vi "AlliGator FMB Run Script.vi"(8 "Error In":errorcluster, 9 "# Steps":i32, 11 "FMB Q Elements in":T18[](array[typedef])) -> (0 "Error Out":errorcluster, 1 "Array of Simulation Outputs":T1[](array[typedef]) {"Simulation & Fit Options & Parameters"."Decay Fit Options & Parameters"."Fit Options"."Confidence Level" min=0.0 max=100.0; "Simulation & Fit Options & Parameters"."Decay Fit Options & Parameters"."Fit Options"."Offset Resolution" min=0.0; "Simulation & Fit Options & Parameters"."Decay Fit Options & Parameters"."Fit Options"."Period" min=0.0; "Simulation & Fit Options & Parameters"."Decay Fit Options & Parameters"."Fit Options"."Min Decay Percentile" min=0.0 max=1.0; "Simulation & Fit Options & Parameters"."Decay Fit Options & Parameters"."Fit Options"."Max Decay Percentile" min=0.0 max=100.0; "Simulation & Fit Options & Parameters"."Decay Fit Options & Parameters"."Fit Parameter Constraints"."Max Value" format="%#.3g"; "Simulation & Fit Options & Parameters"."Decay Fit Options & Parameters"."Fit Parameter Constraints"."Min Value" format="%#.3g"}, 3 "FMB Q Elements out":T18[](array[typedef]), 4 "Message":string)   [LabVIEW 2021, in "AlliGator Fit Method Benchmark.lvlib"]
uses:
  AlliGator Fit Method Benchmark.lvlib
  AlliGator FMB Q Element.ctl
  AlliGator FMB Q Event List.ctl
  Strings/Strings.lvlib
  AlliGator Decay Simulation Parameters.ctl
  AlliGator Fit Simulation Parameters.ctl
  AlliGator Simulation Parameters.ctl
  Fits/Decay Convolution/Decay Model.ctl
  Fits/Fits.lvlib
  Fits/Residual Type.ctl
  Fits/IRF(X)PSED/Fit Weights Type.ctl
  Fits/Non-linear Fitting Method v2.ctl
  Fits/Fit Calculation Method.ctl
  Fits/Non-linear Fitting Algorithm.ctl
  Fits/IRF(X)PSED/Decay Fit Options v3.ctl
  Fits/IRF(X)PSED/Decay Fit Parameters In List.ctl
  Decay Analysis/Decay Fit/AlliGator Decay Fit Parameter Constraints 2.ctl
  Decay Analysis/Decay Fit/AlliGator Decay Fit.lvlib
  Fits/IRF(X)PSED/MLE Baseline Offset Type.ctl
  Decay Fit Parameter Map/AlliGator Decay Fit Options & Parameters v3.ctl
  Decay Fit Parameter Map/AlliGator Decay Fit Parameter Map.lvlib
  AlliGator Simulation & Fit Options & Parameters.ctl
  Arrays/Array Statistics.ctl
  Arrays/Arrays.lvlib
  AlliGator FMB Output.ctl
panel:
  # "see the License on the block diagram (Ctrl+E or Window:Show Block Diagram)"
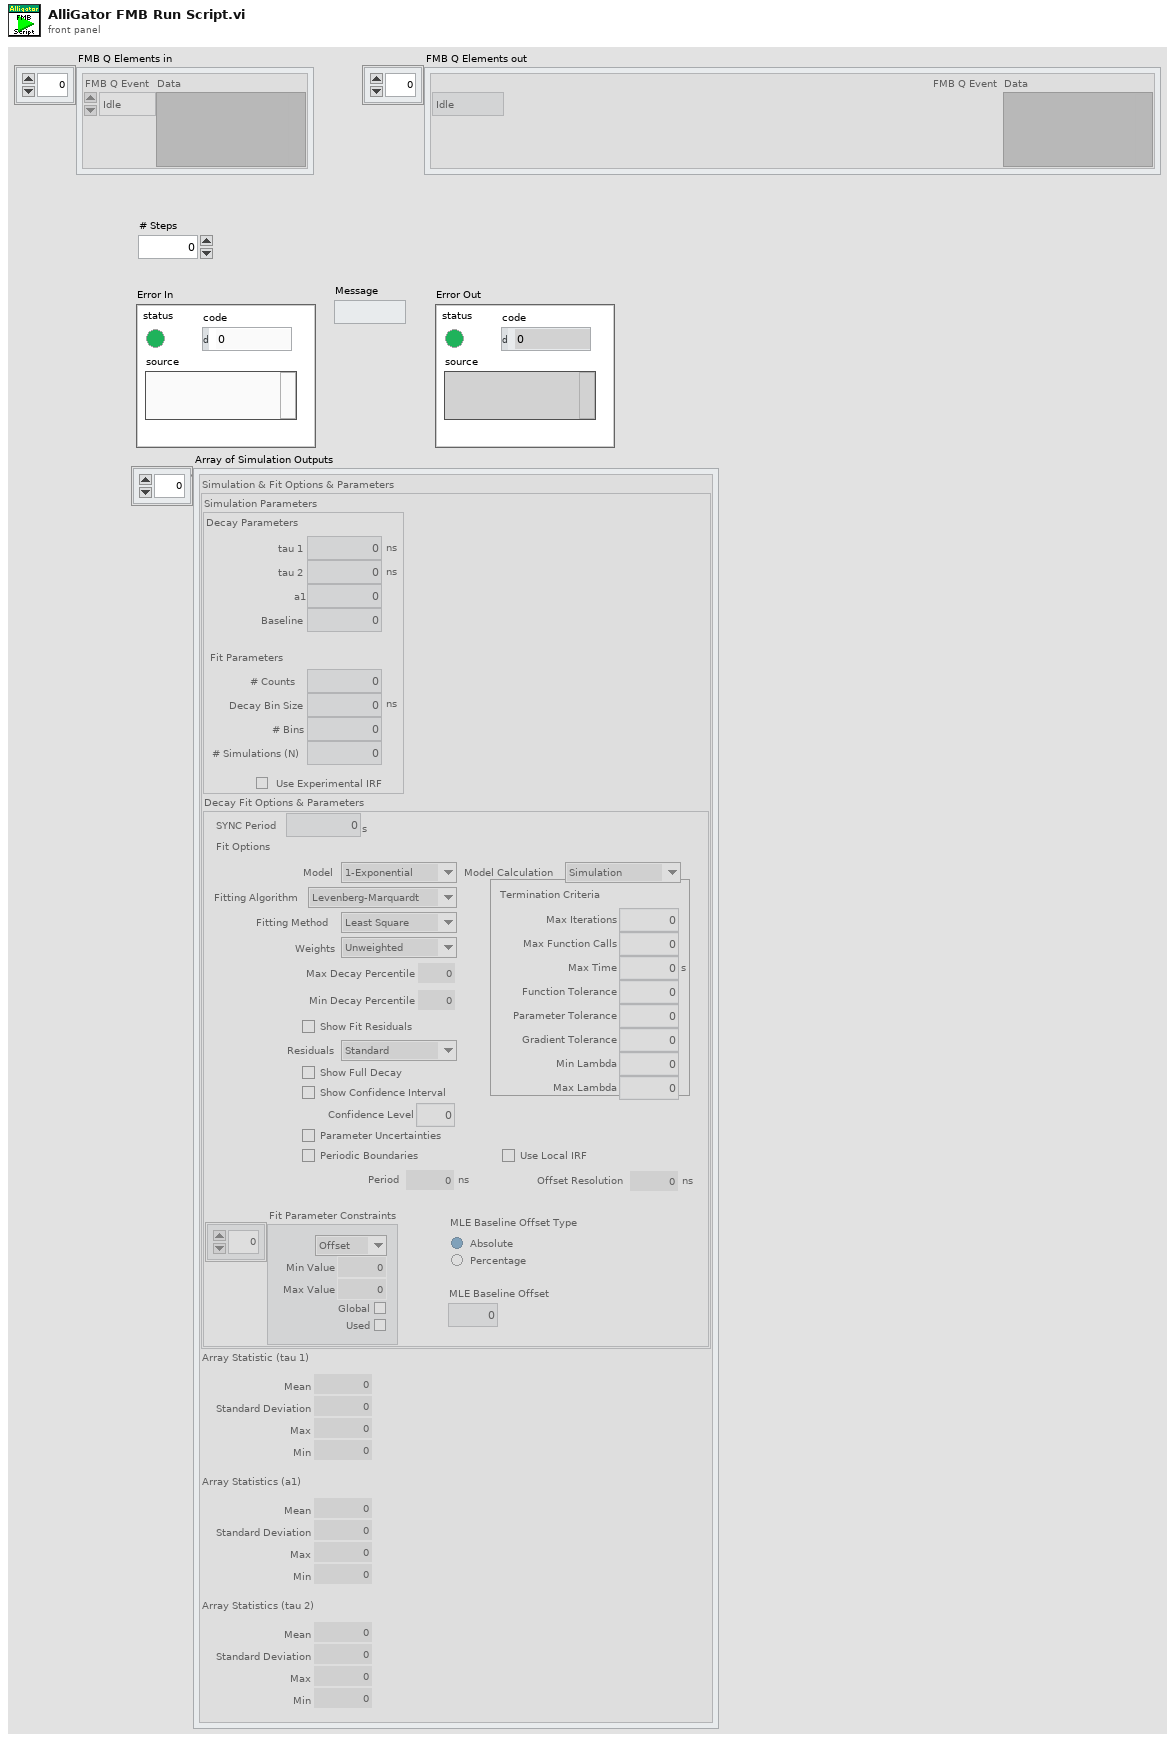
[diagram p1: front panel]
types:
  T1 = typedef "AlliGator Fit Method Benchmark.lvlib/AlliGator FMB Output.ctl" = cluster{"Simulation & Fit Options & Parameters":T2, "Array Statistic (tau 1)":T17, "Array Statistics (a1)":T17, "Array Statistics (tau 2)":T17}
  T2 = typedef "AlliGator Fit Method Benchmark.lvlib/AlliGator Simulation & Fit Options & Parameters.ctl" = cluster{"Simulation Parameters":T3, "Decay Fit Options & Parameters":T6}
  T3 = typedef "AlliGator Fit Method Benchmark.lvlib/AlliGator Simulation Parameters.ctl" = cluster{"Decay Simulation Parameters":T4, "Fit Simulation Parameters":T5, "Use Experimental IRF":bool}
  T4 = typedef "AlliGator Fit Method Benchmark.lvlib/AlliGator Decay Simulation Parameters.ctl" = cluster{"tau 1":dbl[unit], "tau 2":dbl[unit], "a1":dbl, "Baseline":dbl}
  T5 = typedef "AlliGator Fit Method Benchmark.lvlib/AlliGator Fit Simulation Parameters.ctl" = cluster{"# Counts":i32, "# Simulations (N)":i32, "Decay Bin Size":dbl[unit], "# Bins":i32}
  T6 = typedef "AlliGator Decay Fit Parameter Map.lvlib/AlliGator Decay Fit Options & Parameters v3.ctl" = cluster{"SYNC Period":dbl[unit], "Fit Options":T7, "Fit Parameter Constraints":T14[], "MLE Baseline Offset":dbl, "MLE Baseline Offset Type":T16}
  T7 = typedef "Fits.lvlib/Decay Fit Options v3.ctl" = cluster{"Show Fit Residuals":bool, "Fit Model":T8, "Residual Type":T9, "Max Decay Percentile":dbl, "Min Decay Percentile":dbl, "Show Full Decay":bool, "Weights":T10, "Fitting Method":T11, "Compute Parameter Uncertainties":bool, "Periodic Boundaries":bool, "Model Calculation":T12, "Period":dbl[unit], "Termination Criteria":cluster{"Max Iterations":i32, "Max Function Calls":i32, "Max Time":dbl[unit], "Function Tolerance":dbl, "Parameter Tolerance":dbl, "Gradient Tolerance":dbl, "Min Lambda":dbl, "Max Lambda":dbl, "Initial Tick Count":u32}, "Offset Resolution":dbl[unit], "Use Local IRF":bool, "Fitting Algorithm":T13, "Show Confidence Interval ":bool, "Confidence Level":dbl}
  T8 = typedef "Fits.lvlib/Decay Model.ctl" = enum16{"1-Exponential", "2-Exponentials"}
  T9 = typedef "Fits.lvlib/Residual Type.ctl" = enum16{"Standard", "Normalized", "Reduced"}
  T10 = typedef "Fits.lvlib/Fit Weights Type.ctl" = enum16{"Unweighted", "1/Variance", "Best of All"}
  T11 = typedef "Fits.lvlib/Non-linear Fitting Method v2.ctl" = enum16{"Least Square", "Least Absolute Residual", "Bisquare", "MLE", "-", "Best of All"}
  T12 = typedef "Fits.lvlib/Fit Calculation Method.ctl" = enum16{"Simulation", "Convolution", "Integration"}
  T13 = typedef "Fits.lvlib/Non-linear Fitting Algorithm.ctl" = enum16{"Levenberg-Marquardt", "Trust-Region Dogleg"}
  T14 = typedef "AlliGator Decay Fit.lvlib/AlliGator Decay Fit Parameter Constraints 2.ctl" = cluster{"Fit Parameter":T15, "Min Value":dbl, "Max Value":dbl, "Global":bool, "Used":bool}
  T15 = typedef "Fits.lvlib/Decay Fit Parameters In List.ctl" = enum16{"Offset", "Baseline", "A_1", "tau_1", "A_2", "tau_2"}
  T16 = typedef "Fits.lvlib/MLE Baseline Offset Type.ctl" = enum32{"Absolute", "Percentage"}
  T17 = typedef "Arrays.lvlib/Array Statistics.ctl" = cluster{"Mean":dbl, "Standard Deviation":dbl, "Max":dbl, "Min":dbl}
  T18 = typedef "AlliGator Fit Method Benchmark.lvlib/AlliGator FMB Q Element.ctl" = cluster{"FMB Q Event":T19, "Data":variant}
  T19 = typedef "AlliGator Fit Method Benchmark.lvlib/AlliGator FMB Q Event List.ctl" = enum16{"Idle", "Initialization", "Update Script Simulation Parameters", "Single Simulation Prelude", "Run Simulation", "Update Histograms", "Update Script Simulation Output", "Graph Event", "Show Selected Decay", "Export Results", "Update # Processors Used", "Check Baseline", "Run Script", "End Script", "Init", "Abort", "Quit"}
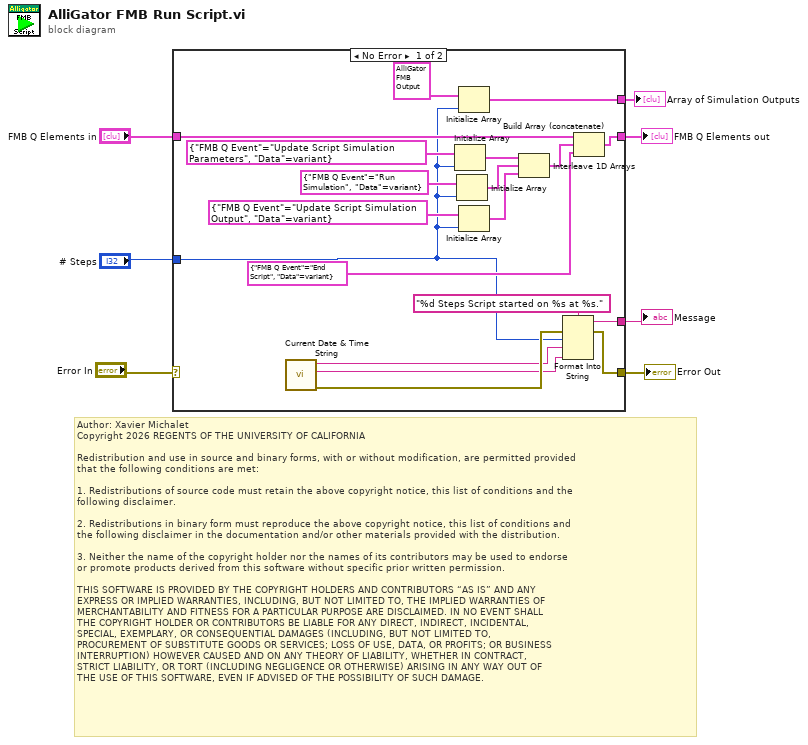
[diagram p0: block diagram]
diagram:
  # "Author: Xavier Michalet\nCopyright 2026 REGENTS OF THE UNIVERSITY OF CALIFORNIA\n\nRedistribution and use in source and binary forms, with or without modification, are permitted provided\nthat the following conditions are met:\n\n1. Redistributions of source code must retain the above copyright notice, this list of conditions and the\nfollowing disclaimer.\n\n2. Redistributions in binary form must reproduce the above copyright notice, this list of conditions and\nthe following disclaimer in the documentation and/or other materials provided with the distribution.\n\n3. Neither the name of the copyright holder nor the names of its contributors may be used to endorse \nor promote products derived from this software without specific prior written permission.\n\nTHIS SOFTWARE IS PROVIDED BY THE COPYRIGHT HOLDERS AND CONTRIBUTORS “AS IS” AND ANY \nEXPRESS OR IMPLIED WARRANTIES, INCLUDING, BUT NOT LIMITED TO, THE IMPLIED WARRANTIES OF\nMERCHANTABILITY AND FITNESS FOR A PARTICULAR PURPOSE ARE DISCLAIMED. IN NO EVENT SHALL\nTHE COPYRIGHT HOLDER OR CONTRIBUTORS BE LIABLE FOR ANY DIRECT, INDIRECT, INCIDENTAL, \nSPECIAL, EXEMPLARY, OR CONSEQUENTIAL DAMAGES (INCLUDING, BUT NOT LIMITED TO, \nPROCUREMENT OF SUBSTITUTE GOODS OR SERVICES; LOSS OF USE, DATA, OR PROFITS; OR BUSINESS\nINTERRUPTION) HOWEVER CAUSED AND ON ANY THEORY OF LIABILITY, WHETHER IN CONTRACT, \nSTRICT LIABILITY, OR TORT (INCLUDING NEGLIGENCE OR OTHERWISE) ARISING IN ANY WAY OUT OF\nTHE USE OF THIS SOFTWARE, EVEN IF ADVISED OF THE POSSIBILITY OF SUCH DAMAGE."
  n1 = case shown="No Error" "Error In" {
    selector: "Error In" -> [_ w28]
    tunnel: "FMB Q Elements in" -> [w26 w27]
    tunnel: [w25 w27] -> w6
    tunnel: "# Steps" -> [w9 _]
    tunnel: [w23 _] -> w4
    tunnel: [w22 w28] -> w3
    tunnel: [w8 _] -> w1
    frame No Error {
      n2 = call "Current Date & Time String.vi"() -> ("Error Out"=w21:errorcluster, "time string"=w19:string, "date string"=w20:string)  [unwired: 9 in]
      n3 = Initialize Array(T18 {"FMB Q Event"=enum."Update Script Simulation Parameters", "Data"=variant} ("FMB Q Elements in"), w9) -> (w24:T18[])
      n4 = Initialize Array(T18 {"FMB Q Event"=enum."Run Simulation", "Data"=variant} ("FMB Q Elements in"), w9) -> (w14:T18[])
      n5 = Initialize Array(T1 {"Simulation & Fit Options & Parameters"={"Simulation Parameters"={"Decay Simulation Parameters"={"tau 1"=0.0, "tau 2"=0.0, "a1"=0.0, "Baseline"=0.0}, "Fit Simulation Parameters"={"# Counts"=0, "# Simulations (N)"=0, "Decay Bin Size"=0.0, "# Bins"=0}, "Use Experimental IRF"=FALSE}, "Decay Fit Options & Parameters"={"SYNC Period"=0.0, "Fit Options"={"Show Fit Residuals"=FALSE, "Fit Model"=enum."1-Exponential", "Residual Type"=enum."Standard", "Max Decay Percentile"=0.0, "Min Decay Percentile"=0.0, "Show Full Decay"=FALSE, "Weights"=enum."Unweighted", "Fitting Method"=enum."Least Square", "Compute Parameter Uncertainties"=FALSE, "Periodic Boundaries"=FALSE, "Model Calculation"=enum."Simulation", "Period"=0.0, "Termination Criteria"={"Max Iterations"=0, "Max Function Calls"=0, "Max Time"=0.0, "Function Tolerance"=0.0, "Parameter Tolerance"=0.0, "Gradient Tolerance"=0.0, "Min Lambda"=0.0, "Max Lambda"=0.0, "Initial Tick Count"=0}, "Offset Resolution"=0.0, "Use Local IRF"=FALSE, "Fitting Algorithm"=enum."Levenberg-Marquardt", "Show Confidence Interval "=FALSE, "Confidence Level"=0.0}, "Fit Parameter Constraints"=[], "MLE Baseline Offset"=0.0, "MLE Baseline Offset Type"=enum."Absolute"}}, "Array Statistic (tau 1)"={"Mean"=0.0, "Standard Deviation"=0.0, "Max"=0.0, "Min"=0.0}, "Array Statistics (a1)"={"Mean"=0.0, "Standard Deviation"=0.0, "Max"=0.0, "Min"=0.0}, "Array Statistics (tau 2)"={"Mean"=0.0, "Standard Deviation"=0.0, "Max"=0.0, "Min"=0.0}} ("Simulation Output"), w9) -> (w8:T1[])
      n6 = Initialize Array(T18 {"FMB Q Event"=enum."Update Script Simulation Output", "Data"=variant} ("FMB Q Elements in"), w9) -> (w11:T18[])
      n7 = Interleave 1D Arrays(w24, w14, w11) -> (w15:T18[])
      n8 = Format Into String(format string="%d Steps Script started on %s at %s.", error in=w21, w9, w20, w19) -> (resulting string=w23:string, error out=w22:errorcluster)  [unwired: 1 in]
      n9 = Build Array (concatenate)(w26, w15, T18 {"FMB Q Event"=enum."End Script", "Data"=variant} ("array")) -> (w25:T18[])
    }
    frame Error {
    }
  }
  "FMB Q Elements out" <- w6
  "Error Out" <- w3
  "Message" <- w4
  "Array of Simulation Outputs" <- w1
